vi "NearestNeighbor.vi"(6 "Algorithm":enum16{"RRT", "A*"}(ring), 7 "target":dbl[](array[numeric]), 8 "k":i32=2, 9 "Depth":i32=1, 10 "index":i32, 11 "KD Tree":dbl[][](array[numeric])) -> ()   [LabVIEW 2016]
uses:
  <vilib>/Analysis/_algsub.llb/Real Vector Norm.vi
  NearestGlobal.vi
  NearestDistanceGlobal.vi
  <vilib>/Analysis/NI_AALPro.lvlib
panel:
  out "error out":errorcluster
  out "path out":path
  in  "error in":errorcluster
  out "Current Dimention":i32
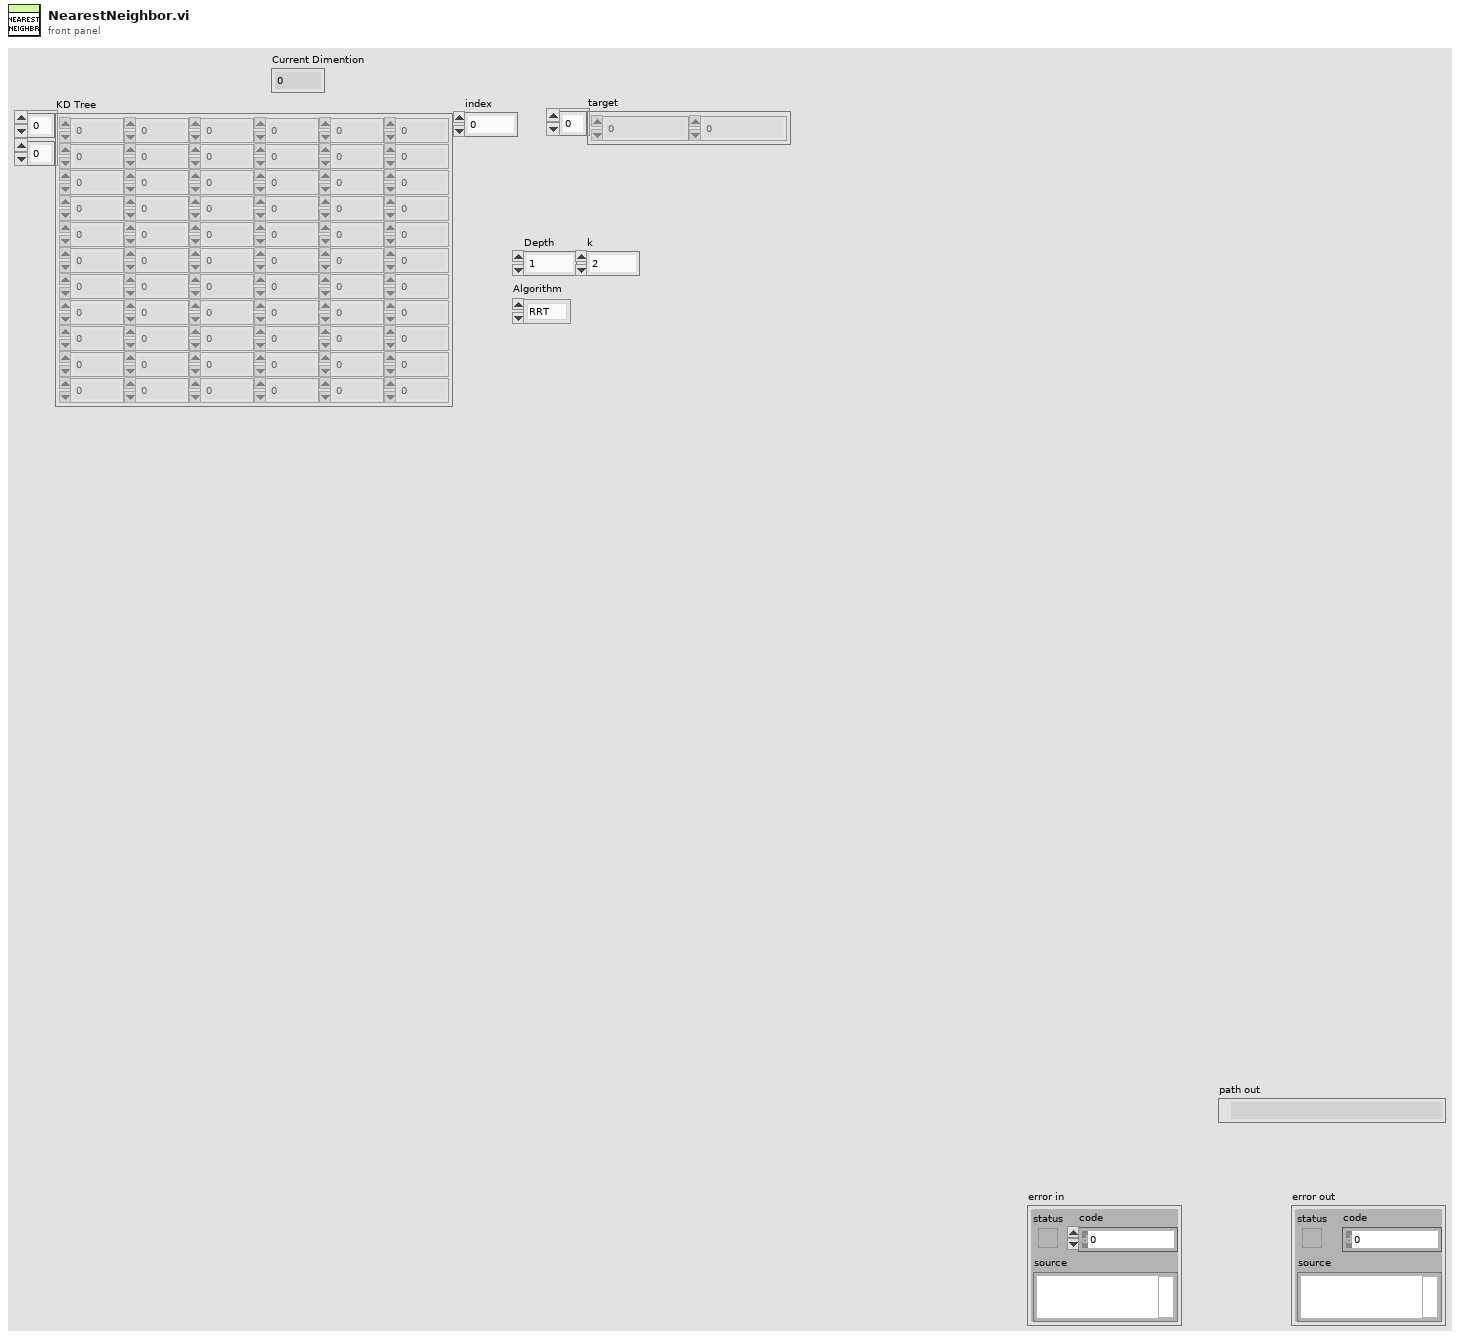
[diagram p1: front panel]
types:
  T1 = enum16{"open", "replace", "create", "open or create", "replace or create", "replace or create with confirmation"}
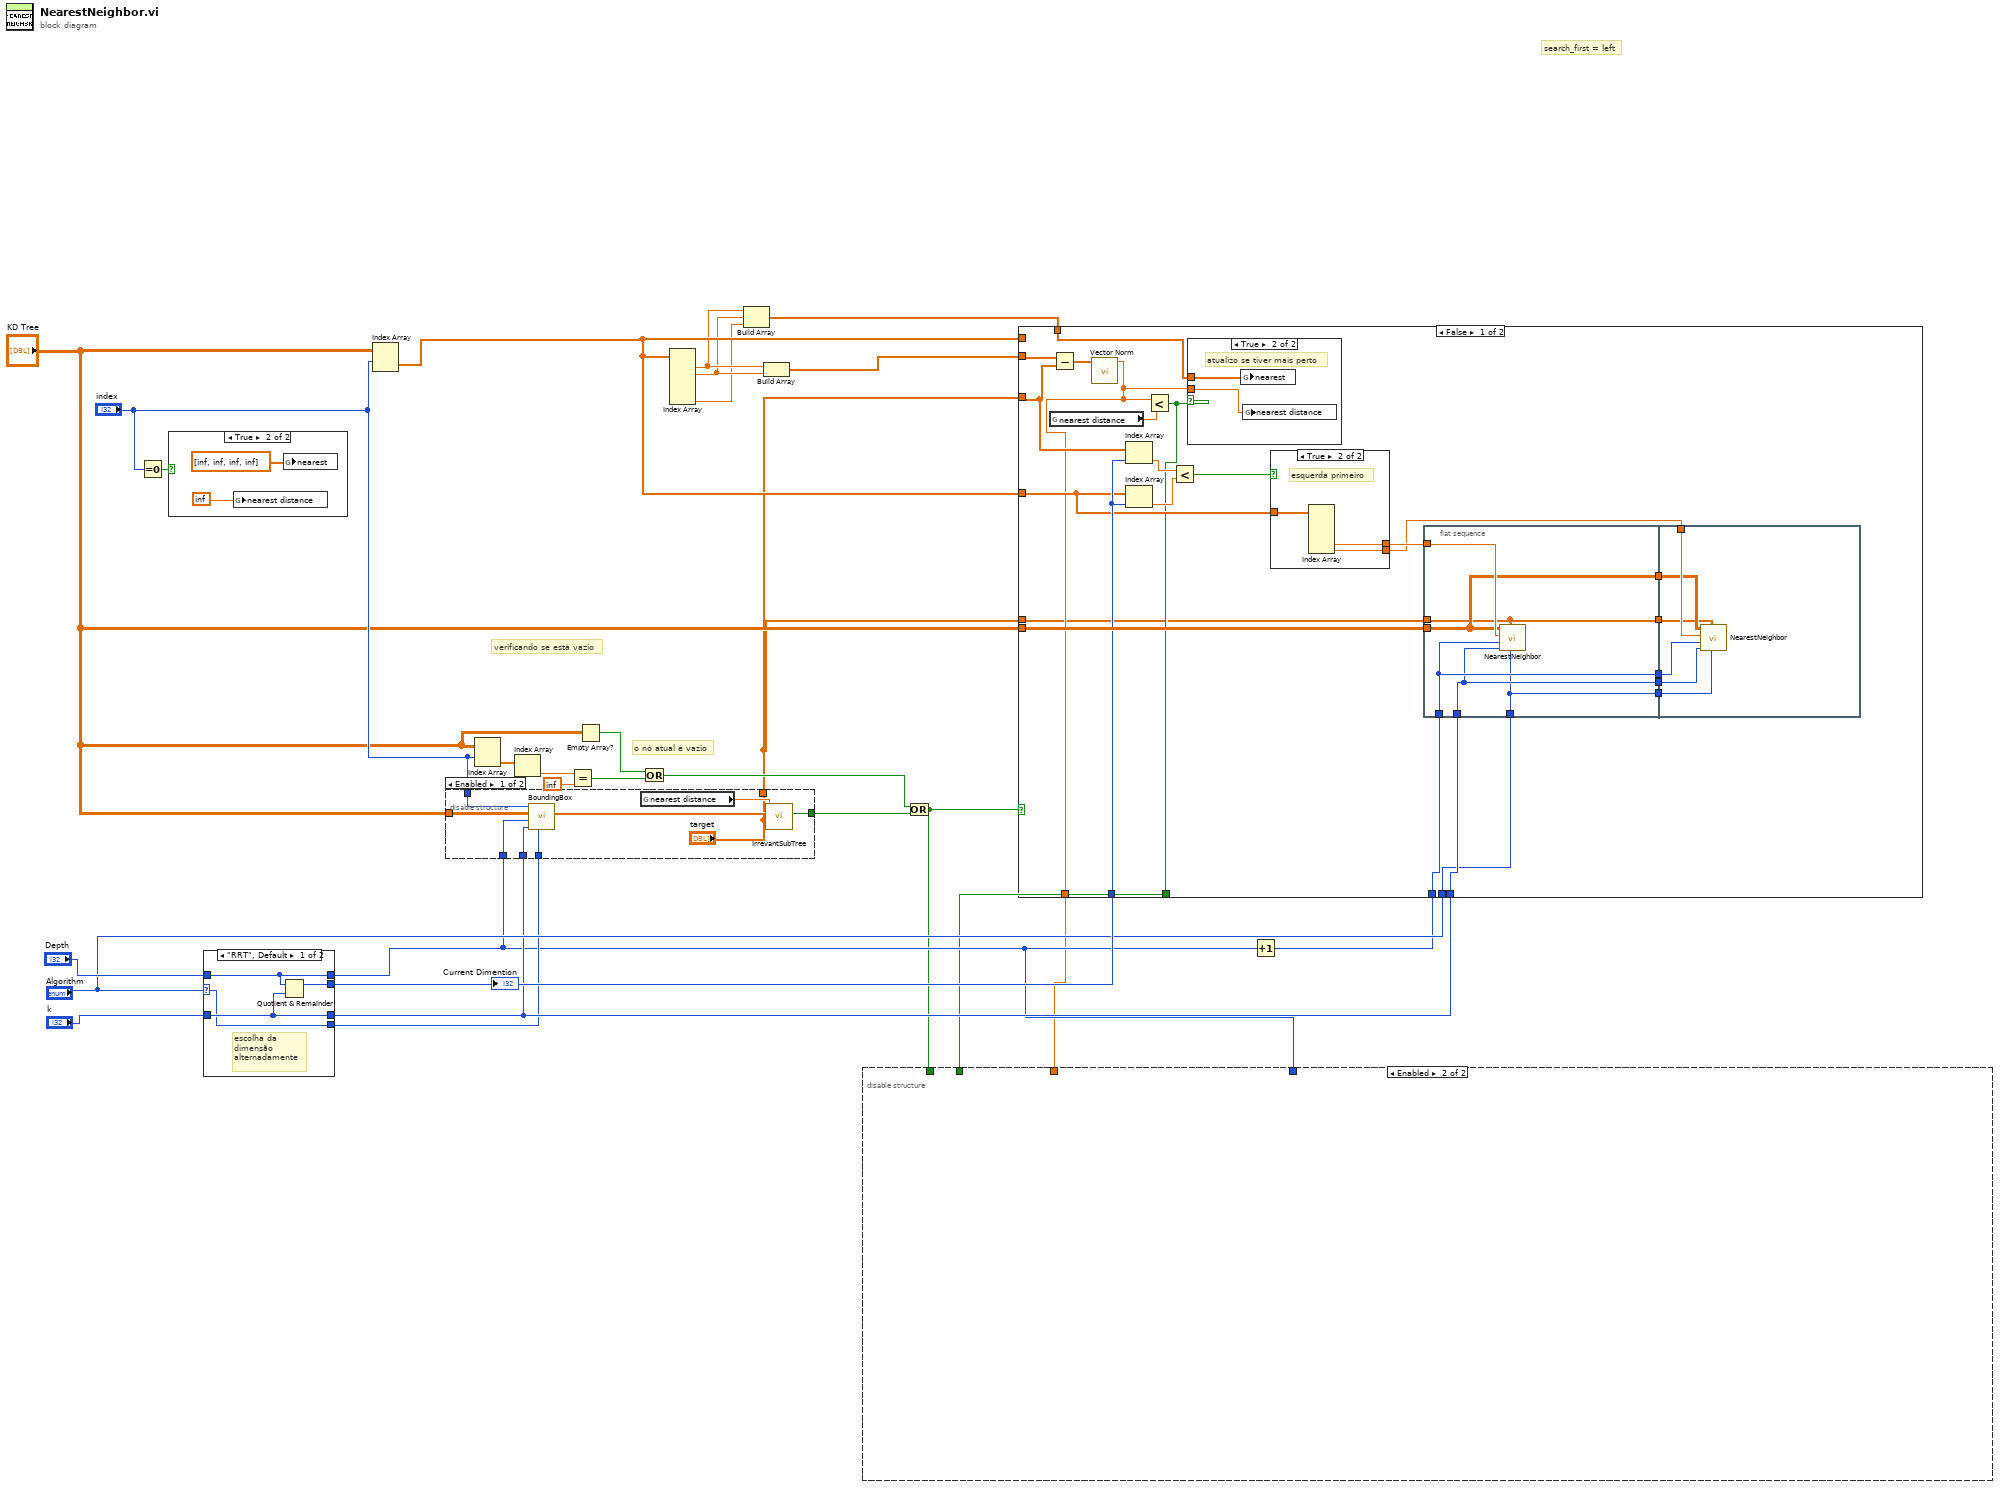
[diagram p0: block diagram]
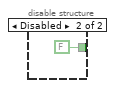
[diagram p2: hidden frame]
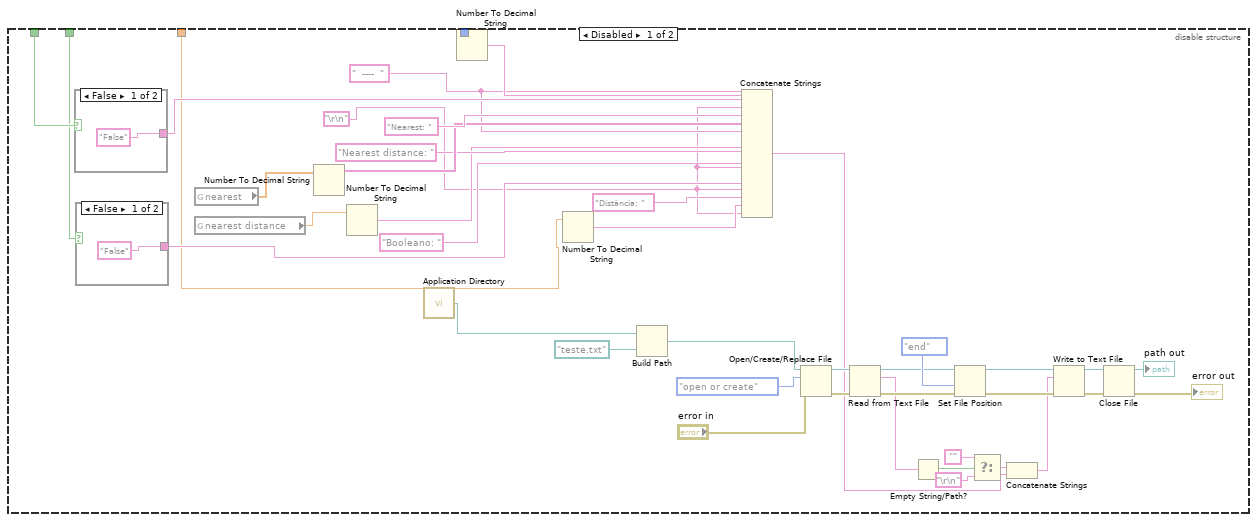
[diagram p3: hidden frame]
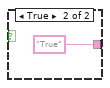
[diagram p4: hidden frame]
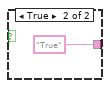
[diagram p5: hidden frame]
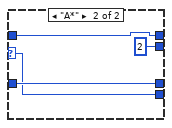
[diagram p7: hidden frame]
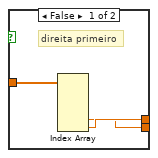
[diagram p8: hidden frame]
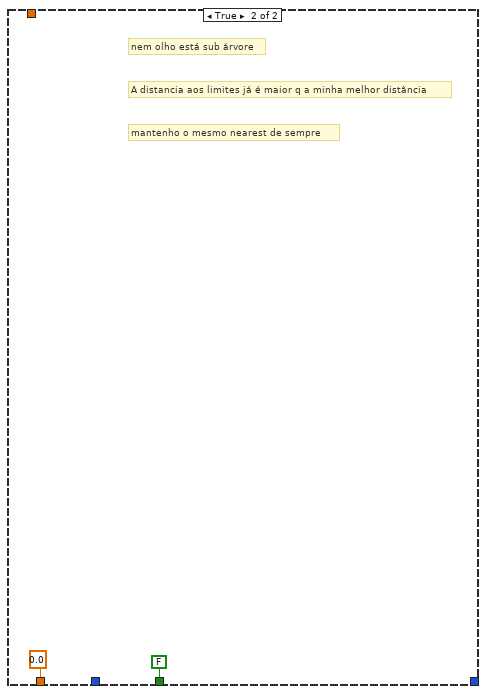
[diagram p10: hidden frame]
diagram:
  # "o nó atual é vazio"
  # "search_first = left"
  # "verificando se está vazio"
  n1 = Equal To 0?(x="index") -> (x = 0?=w14:bool)
  n2 = case shown="True" w14 {
    frame False {
    }
    frame True {
      n3 = global write "NearestDistanceGlobal.vi" "nearest distance"(inf) -> ()
      n4 = global write "NearestGlobal.vi" "nearest"(dbl[] [inf, inf, inf, inf] ("target")) -> ()
    }
  }
  n5 = case shown="\"RRT\", Default" "Algorithm" {
    selector: "Algorithm" -> [w31 w35]
    tunnel: [w34 2] -> w26
    tunnel: [w33 w36] -> w9
    tunnel: [w32 w38] -> w20
    tunnel: "Depth" -> [w33 w36]
    tunnel: "k" -> [w32 w38]
    tunnel: [w31 w35] -> w19
    frame "RRT", Default {
      # "escolha da \ndimensão \nalternadamente"
      n6 = Quotient & Remainder(x=w33, y=w32) -> (x-y*floor(x/y)=w34:i32)  [unwired: 1 out]
    }
    frame "A*" {
    }
  }
  "Current Dimention" <- w26
  n7 = Index Array(array="KD Tree", index (row)="index") -> (element=w16:dbl[])  [unwired: 1 in]
  n8 = disable-structure shown="Enabled" {
    disable-tunnel: w20 -> [w47 _]
    disable-tunnel: w19 -> [w46 _]
    disable-tunnel: [w43 FALSE ("Irrelevant subTree")] -> w15
    disable-tunnel: "index" -> [w42 _]
    disable-tunnel: "KD Tree" -> [w41 _]
    disable-tunnel: w9 -> [w40 _]
    disable-tunnel: ["target" _] -> w5
    frame Enabled {
      n9 = call "BoundingBox.vi"("Algorithm"=w46, "k"=w47, "Depth"=w40, "Tree"=w41, "index"=w42) -> ("Bounding Box"=w44:dbl[])  [unwired: 6 in]
      n10 = global read "NearestDistanceGlobal.vi" "nearest distance"() -> (w45:dbl)
      n11 = call "IrrevantSubTree.vi"("best dist"=w45, "Bounding Box"=w44, "target"="target") -> ("Irrelevant subTree"=w43:bool)  [unwired: 7 in]
    }
    frame Disabled {
    }
  }
  n12 = Index Array(array="KD Tree", index (row)="index") -> (element=w21:dbl[])  [unwired: 1 in]
  n13 = Index Array(array=w21) -> (element=w12:dbl)  [unwired: 1 in]
  n14 = Equal?(x=w12, y=inf) -> (x = y?=w22:bool)
  n15 = Empty Array?(array="KD Tree") -> (empty?=w23:bool)
  n16 = Or(x=w23, y=w22) -> (x .or. y?=w17:bool)
  n17 = Index Array(array=w16) -> (element #1=w4:dbl, element #2=w3:dbl, element #6=w1:dbl)  [unwired: 6 in, 3 out]
  n18 = Build Array(w4, w3, w1) -> (w2:dbl[])
  n19 = Build Array(w4, w3) -> (w18:dbl[])
  n20 = Or(x=w17, y=w15) -> (x .or. y?=w8:bool)
  n21 = Increment(x=w9) -> (x+1=w24:i32)
  n22 = case shown="False" w8 {
    tunnel: w16 -> [_ _]
    tunnel: w26 -> [w67 _]
    tunnel: w24 -> [w60 _]
    tunnel: w20 -> [w57 _]
    tunnel: "Algorithm" -> [w55 _]
    tunnel: w5 -> [w68 _]
    tunnel: w18 -> [w70 _]
    tunnel: "KD Tree" -> [w69 _]
    tunnel: w16 -> [w63 _]
    tunnel: [w53 FALSE] -> w7
    tunnel: [w52 0.0 ("norm")] -> w6
    tunnel: w5 -> [w51 _]
    tunnel: w2 -> [w49 _]
    frame False {
      n23 = global read "NearestDistanceGlobal.vi" "nearest distance"() -> (w71:dbl)
      n24 = Subtract(x=w70, y=w68) -> (x-y=w72:dbl[])
      n25 = call-poly <vilib>:"Vector Norm.vi"("Input Vector"=w72) -> ("norm"=w52:dbl)  [unwired: 9 in, 1 out]
      n26 = Index Array(array=w68, index=w67) -> (element=w66:dbl)
      n27 = Index Array(array=w63, index=w67) -> (element=w65:dbl)
      n28 = Less?(x=w52, y=w71) -> (x < y?=w53:bool)
      n29 = Less?(x=w66, y=w65) -> (x < y?=w64:bool)
      n30 = case shown="True" w53 {
        tunnel: w49 -> [_ w92]
        tunnel: w52 -> [_ w91]
        frame False {
        }
        frame True {
          # "atualizo se tiver mais perto"
          n31 = global write "NearestGlobal.vi" "nearest"(w92) -> ()
          n32 = global write "NearestDistanceGlobal.vi" "nearest distance"(w91) -> ()
        }
      }
      n33 = case shown="True" w64 {
        tunnel: w63 -> [w87 w90]
        tunnel: [w86 w89] -> w62
        tunnel: [w85 w88] -> w61
        frame False {
          # "direita primeiro"
          n34 = Index Array(array=w87) -> (element #4=w85:dbl, element #5=w86:dbl)  [unwired: 5 in, 3 out]
        }
        frame True {
          # "esquerda primeiro"
          n35 = Index Array(array=w90) -> (element #4=w89:dbl, element #5=w88:dbl)  [unwired: 5 in, 3 out]
        }
      }
      n36 = flat-sequence {
        tunnel: w69 -> [w76]
        tunnel: w62 -> [w78]
        tunnel: w60 -> [w77]
        tunnel: [w77] -> w59
        tunnel: [w76] -> w58
        tunnel: w57 -> [w75]
        tunnel: [w75] -> w56
        tunnel: w55 -> [w74]
        tunnel: [w74] -> w54
        tunnel: w51 -> [w73]
        tunnel: [w73] -> w50
        tunnel: w61 -> [w83]
        tunnel: w59 -> [w84]
        tunnel: w58 -> [w82]
        tunnel: w56 -> [w81]
        tunnel: w54 -> [w80]
        tunnel: w50 -> [w79]
        frame #0 {
          n37 = call "NearestNeighbor.vi"("Algorithm"=w74, "target"=w73, "k"=w75, "Depth"=w77, "index"=w78, "KD Tree"=w76) -> ()  [unwired: 6 in]
        }
        frame #1 {
          n38 = call "NearestNeighbor.vi"("Algorithm"=w80, "target"=w79, "k"=w81, "Depth"=w84, "index"=w83, "KD Tree"=w82) -> ()  [unwired: 6 in]
        }
      }
    }
    frame True {
      # "mantenho o mesmo nearest de sempre"
      # "A distancia aos limites já é maior q a minha melhor distância"
      # "nem olho está sub árvore"
    }
  }
  n39 = disable-structure shown="Enabled" {
    disable-tunnel: w9 -> [w135 _]
    disable-tunnel: w8 -> [w133 _]
    disable-tunnel: w7 -> [w100 _]
    disable-tunnel: w6 -> [w97 _]
    frame Disabled {
      w95 = "\r\n"
      w105 = "  ----  " ("string")
      n40 = case shown="False" w133 {
        tunnel: ["False" ("string") "True" ("string")] -> w132
        frame False {
        }
        frame True {
        }
      }
      n41 = case shown="False" w100 {
        tunnel: ["False" ("string") "True" ("string")] -> w99
        frame False {
        }
        frame True {
        }
      }
      n42 = global read "NearestGlobal.vi" "nearest"() -> (w107:dbl[])
      n43 = global read "NearestDistanceGlobal.vi" "nearest distance"() -> (w103:dbl)
      n44 = Number To Decimal String(number=w107) -> (decimal integer string=w106:string[])  [unwired: 1 in]
      n45 = Number To Decimal String(number=w103) -> (decimal integer string=w102:string)  [unwired: 1 in]
      n46 = call <vilib>:"Application Directory.vi"() -> ("Application Directory"=w112:path)
      n47 = Number To Decimal String(number=w135) -> (decimal integer string=w134:string)  [unwired: 1 in]
      n48 = Number To Decimal String(number=w97) -> (decimal integer string=w96:string)  [unwired: 1 in]
      n49 = Build Path(base path=w112, name or relative path=path "teste.txt" ("default name")) -> (appended path=w110:path)
      n50 = Concatenate Strings(w134, w105, w132, w95, "Nearest: " ("string"), w106, w105, "Nearest distance: " ("string"), w102, w95, "Booleano: " ("string"), w99, w95, "Distância: " ("string"), w96, w95) -> (w109:string)
      n51 = Open/Create/Replace File(file path (use dialog)=w110, error in="error in", operation (0:open)=T1."open or create") -> (refnum out=w129:refnum<file>, error out=w128:errorcluster)  [unwired: 3 in, 1 out]
      n52 = Read from Text File(file (use dialog)=w129, error in=w128) -> (refnum out=w123:refnum<file>, text=w117:string, error out=w125:errorcluster)  [unwired: 2 in, 1 out]
      n53 = Empty String/Path?(string/path=w117) -> (empty?=w124:bool)
      n54 = Set File Position(refnum=w123, from (0:start)=enum16{"start", "end", "current"}."end", error in=w125) -> (refnum out=w122:refnum<file>, error out=w121:errorcluster)  [unwired: 1 in]
      n55 = Select(t="", s=w124, f="\r\n") -> (s? t:f=w120:string)
      n56 = Concatenate Strings(w120, w109) -> (w119:string)
      n57 = Write to Text File(file (use dialog)=w122, text=w119, error in=w121) -> (refnum out=w131:refnum<file>, error out=w130:errorcluster)  [unwired: 1 in, 1 out]
      n58 = Close File(refnum=w131, error in=w130) -> (path=→"path out":path, error out=→"error out":errorcluster)
    }
    frame Enabled {
    }
  }
